vi "zmq_join.vi"(3 "error in":errorcluster, 4 "group":string, 5 "socket in":refnum<class "Socket.lvclass">) -> (0 "error out":errorcluster, 2 "socket out":refnum<class "Socket.lvclass">)   [LabVIEW 2025]
doc: "Configure a ZMQ_DISH socket to join the specified group."
uses:
  Socket.lvclass/Socket.ctl
  Socket.lvclass
  ZeroMQ.lvlib
panel:
  # "ØMQ"
  # "labview"
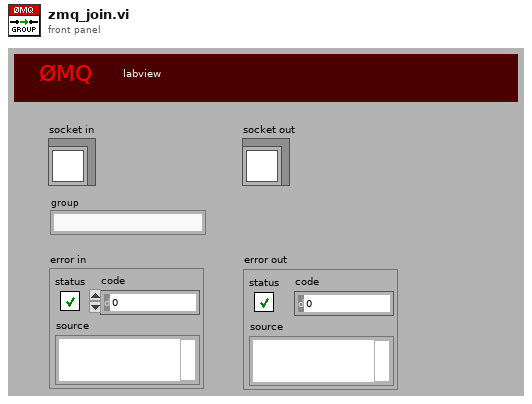
[diagram p1: front panel]
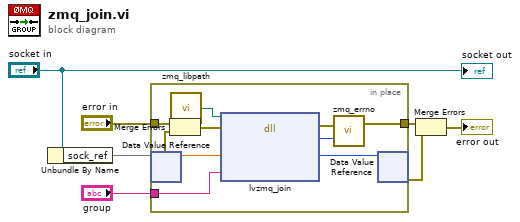
[diagram p0: block diagram]
diagram:
  n1 = Unbundle By Name("socket in") -> ("sock_ref"=w3)
  n2 = in-place {
    in-place-border: "group" -> [w17]
    in-place-border: "error in" -> [w16]
    in-place-border: [w13] -> w5
    n3 = in-place-dvr #1(w3) -> (w12:dbl, w8:errorcluster)
    n4 = Merge Errors(w16, w8) -> (w9:errorcluster)
    n5 = call "zmq_libpath.vi"() -> ("path"=w10:path)
    n6 = dll-call lib="?" fn="lvzmq_join" ("zmq_labview.dll:lvzmq_bind")(path in=w10, error in=w9, "sock_obj"=w12, "group"=w17) -> (error out=w15:errorcluster, "return type"=w14:i32, "sock_obj"=w11:u64)  [unwired: 2 in, 1 out]
    n7 = call "zmq_errno.vi"("retval"=w14, "error in"=w15) -> ("error out"=w13:errorcluster)  [unwired: 1 out]
    n8 = in-place-dvr #1(w11) -> (w1:errorcluster)  [unwired: 1 out]
  }
  n9 = Merge Errors(w5, w1) -> (→"error out":errorcluster)
  "socket out" <- "socket in"
